vi "Main.vi"(11 "Module Admin":refnum<class "Delacor_lib_QMH_Module Admin.lvclass">) -> ()   [LabVIEW 2024, in "Aggregation 1.lvlib"]
doc: "This template is based off of the Queued Message Handler design pattern and the Queued Message Handler project template that ships with LabVIEW.\n\nThe main difference is that the queue is private to this module and communication between modules is performed via Broadcast and Request events.\n\nRequest events are wrapped in public API methods and are handled in the Event Handling Loop (EHL) of this VI. Any module can register for Broadcast events sent by this module. The EHL generates messages based on user interface actions.\n\nThe Message Handling Loop (MHL) processes messages generated by the EHL, or by other messages. The messages are string values, so new messages can be added easily to the Message Cases case structure in the MHL. Each message cluster can also provide an optional value for Message Data, which is a variant that can be converted to whatever message-specific data is required.\n_____\nBased on DQMH Dev Tools: Project Template 7.1.0.1503."
uses:
  Aggregation 1.lvlib
  <vilib>/Delacor/Delacor QMH/Libraries/Module Admin_class/Delacor_lib_QMH_Module Admin.lvclass
  Controls/Agg level 1 state cluster.ctl
  Controls/Agg level 1 state enum.ctl
  Module Data--cluster.ctl
  <vilib>/Delacor/Delacor QMH/Libraries/Message Queue_class/Delacor_lib_QMH_Message Queue.lvclass/Delacor_lib_QMH_Message Queue.ctl
  Stop Argument--cluster.ctl
  <vilib>/Delacor/Delacor QMH/Libraries/Module Admin_class/Delacor_lib_QMH_Module Admin.lvclass/Delacor_lib_QMH_Module Admin.ctl
  Serial received Argument--cluster.ctl
  Level completed Argument--cluster.ctl
  <vilib>/Utility/miscctls.llb/LVPointTypeDef.ctl
  <vilib>/Delacor/Delacor QMH/Libraries/Message Queue_class/Delacor_lib_QMH_Enqueue Message (Single).vi
  <vilib>/Delacor/Delacor QMH/Libraries/Module Admin_class/Delacor_lib_QMH_Get External Launch.vi
  <vilib>/Delacor/Delacor QMH/Libraries/Message Queue_class/Delacor_lib_QMH_Message Queue.lvclass
  DB/DB.lvlib
  GUI/GUI.lvlib
panel:
  out "error out":errorcluster
  out "Status":string
  in  "Simulate MHL Error":bool
  in  "Simulate EHL Error":bool
  # "Other processes communicate with this Module via its Public API (wrappers for its Request Events).\n\nThis Module communicates with other processes via its Broadcast Events.\nAny process that wants to receive these messages can register for this module's Broadcast events."
  # "This template is for the DQMH framework. See the block diagram for more information on how to use this template."
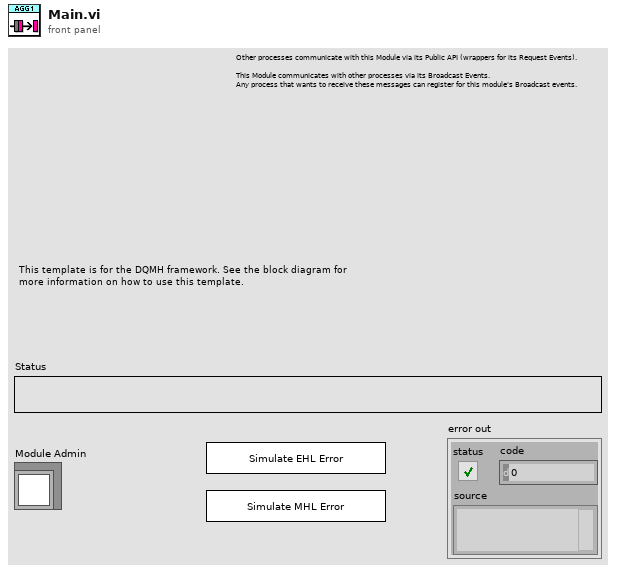
[diagram p1: front panel]
types:
  T1 = typedef "Agg level 1 state cluster.ctl" = cluster{"State":T2, "Data":variant}
  T2 = typedef "Agg level 1 state enum.ctl" = enum16{"init", "counting children", "level completed", "parent ready", "parent linked", "error", "terminate"}
  T3 = typedef "Aggregation 1.lvlib/Request Events--cluster.ctl" = cluster{"Stop Module":refnum<user-event>, "Show Panel":refnum<user-event>, "Hide Panel":refnum<user-event>, "Get Module Execution Status":refnum<user-event>, "Show Diagram":refnum<user-event>, "Serial received":refnum<user-event>, "Level completed":refnum<user-event>}
  T4 = typedef "Aggregation 1.lvlib/Module Data--cluster.ctl" = cluster{"Status":string}
  T5 = enum32{"invalid lock state", "Not Locked", "Locked (No Password)", "Password-protected"}
  T6 = typedef "Aggregation 1.lvlib/Stop Argument--cluster.ctl" = cluster{"Origin":string, "Exit via Stop Module Req?":bool, "Wait for Module to stop?":bool}
  T7 = typedef "Aggregation 1.lvlib/Serial received Argument--cluster.ctl" = cluster{"Serial":string, "index":dbl}
  T8 = typedef "Aggregation 1.lvlib/Level completed Argument--cluster.ctl" = cluster{"Serial array":string[], "Level":dbl}
  T9 = typedef "LVPointTypeDef.ctl" = cluster{"Horizontal":i16, "Vertical":i16}
  T10 = enum32{"Invalid", "Standard", "Closed", "Hidden", "Minimized", "Maximized"}
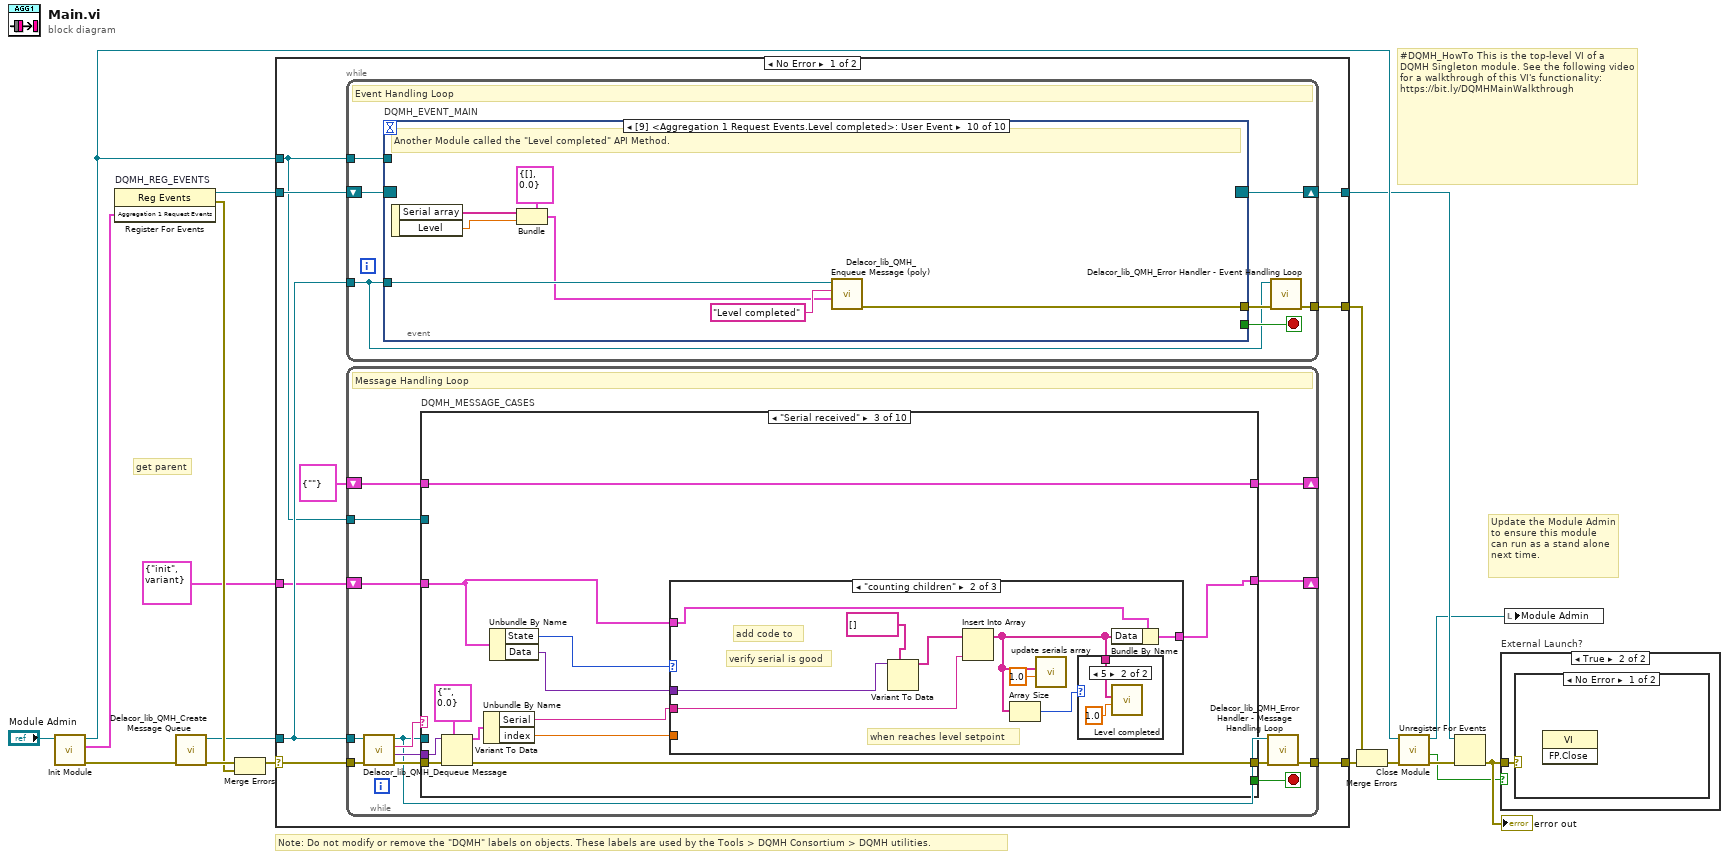
[diagram p0: block diagram]
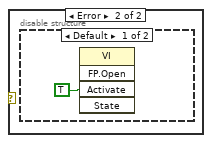
[diagram p3: hidden frame]
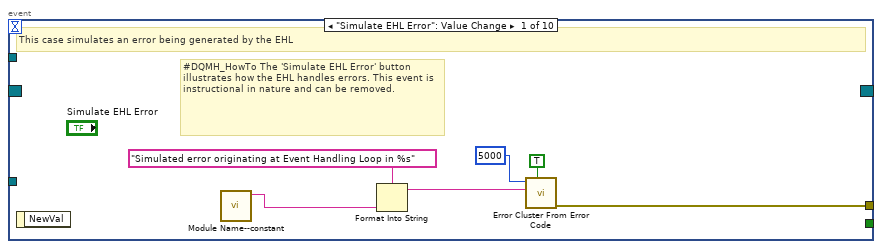
[diagram p5: hidden frame]
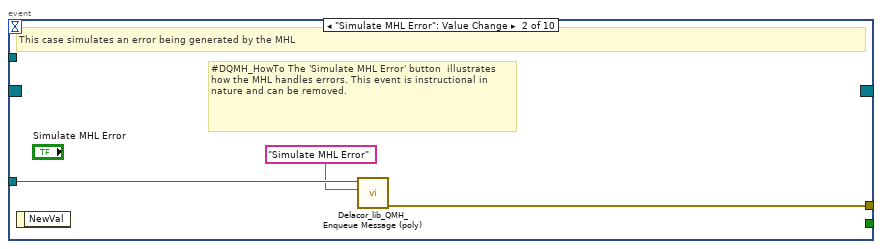
[diagram p6: hidden frame]
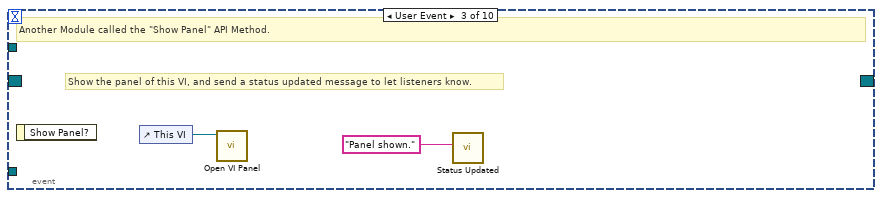
[diagram p7: hidden frame]
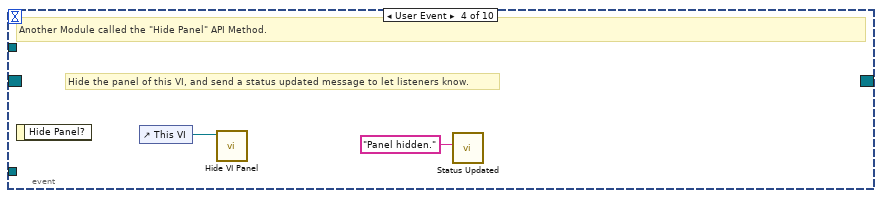
[diagram p8: hidden frame]
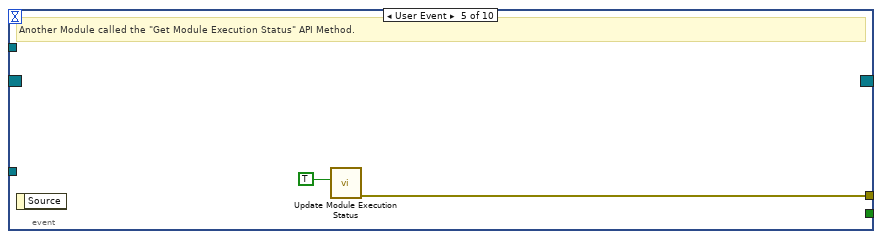
[diagram p9: hidden frame]
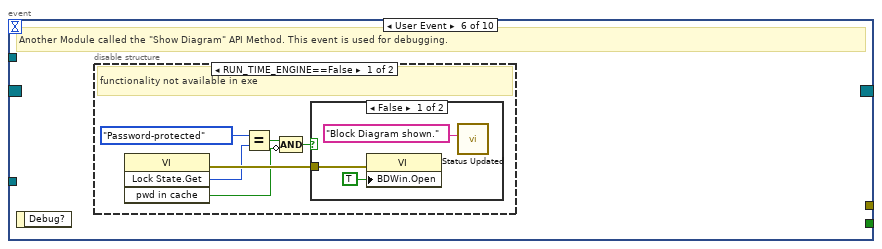
[diagram p10: hidden frame]
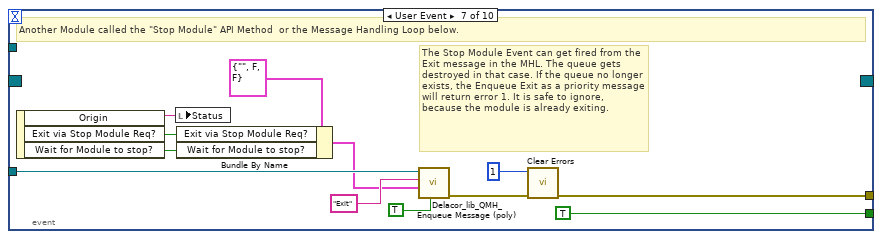
[diagram p13: hidden frame]
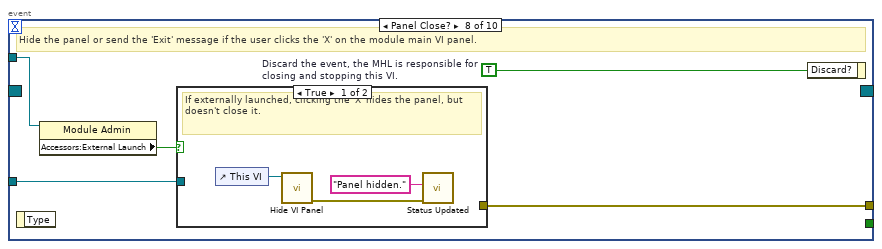
[diagram p14: hidden frame]
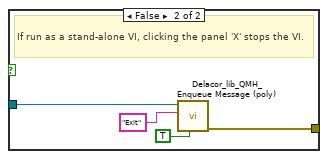
[diagram p15: hidden frame]
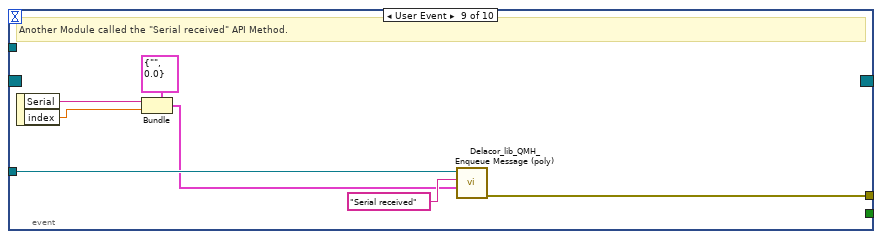
[diagram p16: hidden frame]
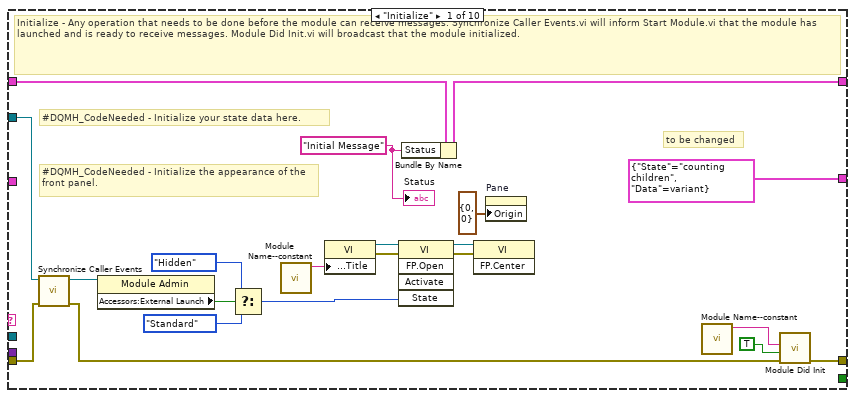
[diagram p17: hidden frame]
diagram:
  # "get parent"
  # "#DQMH_HowTo This is the top-level VI of a DQMH Singleton module. See the following video for a walkthrough of this VI's functionality: https://bit.ly/DQMHMainWalkthrough"
  # "Note: Do not modify or remove the \"DQMH\" labels on objects. These labels are used by the Tools > DQMH Consortium > DQMH utilities."
  # "Update the Module Admin to ensure this module can run as a stand alone next time."
  n1 = call "Init Module.vi"("Singleton Module Admin in"="Module Admin") -> ("error out"=w17:errorcluster, "Aggregation 1 Request Events"=w6:T3, "Singleton Module Admin out"=w9:refnum<class "Delacor_lib_QMH_Module Admin.lvclass">)  [unwired: 8 in]
  n2 = register-events "DQMH_REG_EVENTS"(w6) -> (reference out=w7:refnum<event-registration>, error out=w10:errorcluster)  [unwired: 2 in]
  n3 = call <vilib>:"Delacor_lib_QMH_Create Message Queue.vi"("error in"=w17) -> ("error out"=w12:errorcluster, "Message Queue"=w5:refnum<class "Delacor_lib_QMH_Message Queue.lvclass">)  [unwired: 9 in]
  n4 = Merge Errors(w12, w10) -> (w11:errorcluster)
  n5 = case shown="No Error" w11 {
    selector: w11 -> [w25 w248]
    tunnel: [w27 w247] -> w18
    tunnel: [w24 w246] -> w8
    tunnel: w7 -> [w22 w246]
    tunnel: w5 -> [w21 w241]
    tunnel: [w26 _] -> w15
    tunnel: w9 -> [w20 w242]
    tunnel: T1 {"State"=enum."init", "Data"=variant(dbl 0.0)} -> [w19 _]
    frame No Error {
      n6 = while {
        tunnel: w21 -> [w28]
        shift-right: [w31] -> w24
        shift-left: w22 -> [w32]
        tunnel: [w33] -> w26
        tunnel: w20 -> [w29]
        stop <- w30 stop-if-true
        # "Event Handling Loop"
        n7 = event "DQMH_EVENT_MAIN" shown="[9] <Aggregation 1 Request Events.Level completed>: User Event" {
          selector: w32 -> [_ _ _ _ _ _ _ _ _ _]
          dyn-events: [_ _ _ _ _ _ _ _ _ _] -> w31
          timeout: _ -> [_ _ _ _ _ _ _ _ _ _]
          tunnel: [_ _ _ _ _ _ TRUE ("Discard?") _ _ _] -> w30
          tunnel: w28 -> [_ w42 _ _ _ _ w66 w73 w89 w96]
          tunnel: [w40 w43 _ _ w49 _ w69 w75 w83 w90] -> w34
          tunnel: w29 -> [_ _ _ _ _ _ _ w72 _ _]
          event "Simulate EHL Error": Value Change {
            # "#DQMH_HowTo The 'Simulate EHL Error' button  illustrates how the EHL handles errors. This event is instructional in nature and can be removed."
            # "This case simulates an error being generated by the EHL"
            n8 = event-data() -> ()  [unwired: 1 in, 1 out]
            n9 = call "Module Name--constant.vi"() -> ("Module Name"=w37:string)  [unwired: 11 in]
            n10 = Format Into String(format string="Simulated error originating at Event Handling Loop in %s", w37) -> (resulting string=w38:string)  [unwired: 2 in, 1 out]
            n11 = call <vilib>:"Error Cluster From Error Code.vi"("show call chain? (False)"=TRUE, "error message (\"\")"=w38, "error code (0)"=5000) -> ("error out"=w40:errorcluster)  [unwired: 6 in]
          }
          event "Simulate MHL Error": Value Change {
            # "#DQMH_HowTo The 'Simulate MHL Error' button  illustrates how the MHL handles errors. This event is instructional in nature and can be removed."
            # "This case simulates an error being generated by the MHL"
            n12 = event-data() -> ()  [unwired: 1 in, 1 out]
            n13 = call-poly <vilib>:"Delacor_lib_QMH_Enqueue Message (poly).vi"("Message"="Simulate MHL Error", "Message Queue in"=w42) -> ("error out"=w43:errorcluster)  [unwired: 8 in, 1 out]
          }
          event User Event {
            # "Show the panel of this VI, and send a status updated message to let listeners know."
            # "Another Module called the \"Show Panel\" API Method."
            n14 = event-data() -> ()  [unwired: 1 in, 1 out]
            n15 = control-ref of="This VI"() -> (w45:refnum<vi>)
            n16 = call "Open VI Panel.vi"("VI"=w45) -> ()  [unwired: 10 in, 1 out]
            n17 = call "Status Updated.vi"("Status"="Panel shown." ("format string")) -> ()  [unwired: 10 in, 1 out]
          }
          event User Event {
            # "Hide the panel of this VI, and send a status updated message to let listeners know."
            # "Another Module called the \"Hide Panel\" API Method."
            n18 = event-data() -> ()  [unwired: 1 in, 1 out]
            n19 = control-ref of="This VI"() -> (w47:refnum<vi>)
            n20 = call "Hide VI Panel.vi"("VI"=w47) -> ()  [unwired: 10 in, 1 out]
            n21 = call "Status Updated.vi"("Status"="Panel hidden." ("format string")) -> ()  [unwired: 10 in, 1 out]
          }
          event User Event {
            # "Another Module called the \"Get Module Execution Status\" API Method."
            n22 = event-data() -> ()  [unwired: 1 in, 1 out]
            n23 = call "Update Module Execution Status.vi"("Running?"=TRUE) -> ("error out"=w49:errorcluster)  [unwired: 10 in]
          }
          event User Event {
            # "Another Module called the \"Show Diagram\" API Method. This event is used for debugging."
            n24 = event-data() -> ()  [unwired: 1 in, 1 out]
            n25 = disable-structure shown="RUN_TIME_ENGINE==False" {
              frame condition #0 (active) {
                # "functionality not available in exe"
                n26 = invoke on="Invoke Node" class="VI" method="Lock State.Get"() -> (error out=w55:errorcluster, "Get Lock State"=w54:T5, "pwd in cache"=w51:bool)  [unwired: 4 in, 1 out]
                n27 = Equal?(x=T5."Password-protected", y=w54) -> (x = y?=w52:bool)
                n28 = Compound Arithmetic op=AND(w52, invert w51) -> (w50:bool)
                n29 = case shown="False" w50 {
                  tunnel: w55 -> [w58 _]
                  frame False {
                    n30 = property on="Property Node" class="VI"(error in=w58, "BDWin.Open"=TRUE ("Block Diagram Window:Open")) -> ()  [unwired: 1 in, 2 out]
                    n31 = call "Status Updated.vi"("Status"="Block Diagram shown." ("format string")) -> ()  [unwired: 10 in, 1 out]
                  }
                  frame True {
                    # "Password-protected VI, and the password is not in the cache. Do not show the diagram."
                  }
                }
              }
              frame condition #1 {
              }
            }
          }
          event User Event {
            # "The Stop Module Event can get fired from the Exit message in the MHL. The queue gets destroyed in that case. If the queue no longer exists, the Enqueue Exit as a priority message will return error 1. It is safe to ignore, because the module is already exiting."
            # "Another Module called the \"Stop Module\" API Method  or the Message Handling Loop below."
            n32 = event-data() -> ("Origin"=w65:string, "Exit via Stop Module Req?"=w61:bool, "Wait for Module to stop?"=w60:bool)  [unwired: 1 in]
            n33 = local write "Status"(w65) -> ()
            n34 = Bundle By Name(cluster=T6 {"Origin"="", "Exit via Stop Module Req?"=FALSE, "Wait for Module to stop?"=FALSE} ("Stop Argument"), "Exit via Stop Module Req?"=w61, "Wait for Module to stop?"=w60) -> (w59:T6)
            n35 = call-poly <vilib>:"Delacor_lib_QMH_Enqueue Message (poly).vi"("Priority Message? (F)"=TRUE, "Message Data"=w59, "Message"="Exit", "Message Queue in"=w66) -> ("error out"=w70:errorcluster)  [unwired: 6 in, 1 out]
            n36 = call <vilib>:"Clear Errors.vi"("error in (no error)"=w70, "specific error code to clear (0: all)"=1) -> ("error out"=w69:errorcluster)  [unwired: 4 in, 1 out]
          }
          event Panel Close? {
            w74 = TRUE  # Discard the event, the MHL is responsible for closing and stopping this VI.
            # "Hide the panel or send the 'Exit' message if the user clicks the 'X' on the module main VI panel."
            n37 = event-data() -> ()  [unwired: 1 in, 1 out]
            n38 = property on="Property Node" class="Module Admin"(reference=w72) -> ("Accessors:External Launch"=w71:bool)  [unwired: 1 in, 2 out]
            n39 = case shown="True" w71 {
              tunnel: w73 -> [_ w81]
              tunnel: [_ w82] -> w75
              frame True {
                # "If externally launched, clicking the 'X' hides the panel, but doesn't close it."
                n40 = control-ref of="This VI"() -> (w78:refnum<vi>)
                n41 = call "Hide VI Panel.vi"("VI"=w78) -> ("error out"=w76:errorcluster)  [unwired: 10 in]
                n42 = call "Status Updated.vi"("error in"=w76, "Status"="Panel hidden." ("format string")) -> ()  [unwired: 9 in, 1 out]
              }
              frame False {
                # "If run as a stand-alone VI, clicking the panel 'X' stops the VI."
                n43 = call-poly <vilib>:"Delacor_lib_QMH_Enqueue Message (poly).vi"("Priority Message? (F)"=TRUE, "Message"="Exit", "Message Queue in"=w81) -> ("error out"=w82:errorcluster)  [unwired: 7 in, 1 out]
              }
            }
            n44 = event-data ("Event Filter Node")("Discard?"=w74) -> ()  [unwired: 1 in, 1 out]
          }
          event User Event {
            # "Another Module called the \"Serial received\" API Method."
            n45 = event-data() -> ("Serial"=w85:string, "index"=w84:dbl)  [unwired: 1 in]
            n46 = Bundle(cluster=T7 {"Serial"="", "index"=0.0} ("Serial received Argument"), "Serial"=w85, "index"=w84) -> (w86:T7)
            n47 = call-poly <vilib>:"Delacor_lib_QMH_Enqueue Message (poly).vi"("Message Data"=w86, "Message"="Serial received", "Message Queue in"=w89) -> ("error out"=w83:errorcluster)  [unwired: 7 in, 1 out]
          }
          event User Event {
            # "Another Module called the \"Level completed\" API Method."
            n48 = event-data() -> ("Serial array"=w92:string[], "Level"=w91:dbl)  [unwired: 1 in]
            n49 = Bundle(cluster=T8 {"Serial array"=[], "Level"=0.0} ("Level completed Argument"), "Serial array"=w92, "Level"=w91) -> (w93:T8)
            n50 = call-poly <vilib>:"Delacor_lib_QMH_Enqueue Message (poly).vi"("Message Data"=w93, "Message"="Level completed", "Message Queue in"=w96) -> ("error out"=w90:errorcluster)  [unwired: 7 in, 1 out]
          }
        }
        n51 = call-dynamic "Delacor_lib_QMH_Error Handler - Event Handling Loop.vi"("error in"=w34, "Message Queue in"=w28) -> ("dup error in"=w33:errorcluster)  [unwired: 8 in, 1 out]
      }
      n52 = while {
        tunnel: w21 -> [w99]
        shift-right: [w107] -> _
        shift-left: T4 {"Status"=""} ("Data Cluster") -> [w108]
        tunnel: w25 -> [w110]
        tunnel: [w102] -> w27
        tunnel: w20 -> [w103]
        shift-right: [w97] -> _
        shift-left: w19 -> [w98]
        stop <- w106 stop-if-true
        # "Message Handling Loop"
        n53 = call-dynamic "Delacor_lib_QMH_Dequeue Message.vi"("error in"=w110, "Message Queue in"=w99) -> ("error out"=w109:errorcluster, "Message Data"=w104:variant, "Message"=w105:string, "Message Queue out"=w100:refnum<class "Delacor_lib_QMH_Message Queue.lvclass">)  [unwired: 6 in]
        n54 = case "DQMH_MESSAGE_CASES" shown="\"Serial received\"" w105 {
          selector: w105 -> [_ _ _ _ _ _ _ _ _ w236]
          tunnel: w100 -> [_ _ _ _ _ _ _ w200 w223 _]
          tunnel: w109 -> [w129 w134 w146 w173 w182 w185 w195 w207 w229 w239]
          tunnel: [w127 w134 w144 w171 w181 w185 w194 w203 w224 w240] -> w101
          tunnel: w108 -> [w118 w133 w145 w172 w180 w184 w192 w202 w222 w237]
          tunnel: [w117 w133 w145 w172 w180 w184 w192 w202 w222 w237] -> w107
          tunnel: [_ _ _ _ _ _ _ _ w221 _] -> w106
          tunnel: w104 -> [_ _ w143 w170 _ _ _ w201 w220 _]
          tunnel: w103 -> [w119 _ _ _ _ _ _ w199 w215 _]
          tunnel: w98 -> [_ w132 w135 w160 w179 w183 w186 w196 w214 w230]
          tunnel: [T1 {"State"=enum."counting children", "Data"=variant} w132 w136 w161 w179 w183 w186 w196 w214 w230] -> w97
          frame "Initialize" {
            w113 = "Initial Message" ("Initial Message")
            # "to be changed"
            # "#DQMH_CodeNeeded - Initialize the appearance of the front panel."
            # "#DQMH_CodeNeeded - Initialize your state data here."
            # "Initialize - Any operation that needs to be done before the module can receive messages. Synchronize Caller Events.vi will inform Start Module.vi that the module has launched and is ready to receive messages. Module Did Init.vi will broadcast that the module initialized."
            n55 = call "Synchronize Caller Events.vi"("error in"=w129, "Singleton Module Admin in"=w119) -> ("error out"=w128:errorcluster, "Singleton Module Admin out"=w114:refnum<class "Delacor_lib_QMH_Module Admin.lvclass">)  [unwired: 8 in]
            n56 = property on="Property Node" class="Module Admin"(reference=w114) -> ("Accessors:External Launch"=w123:bool)  [unwired: 1 in, 2 out]
            n57 = Select(t=T10."Hidden" ("State"), s=w123, f=T10."Standard" ("State")) -> (s? t:f=w120:T10)
            n58 = call "Module Name--constant.vi"() -> ("Module Name"=w126:string)  [unwired: 11 in]
            n59 = property on="Property Node" class="VI"("Front Panel.Title"=w126) -> (reference out=w125:refnum<vi>, error out=w131:errorcluster)  [unwired: 2 in]
            n60 = invoke on="Invoke Node" class="VI" method="FP.Open"(reference=w125, error in=w131, "State"=w120) -> (reference out=w124:refnum<vi>, error out=w130:errorcluster)  [unwired: 2 in, 3 out]
            n61 = Bundle By Name(cluster=w118, "Status"=w113) -> (w117:T4)
            n62 = invoke on="Invoke Node" class="VI" method="FP.Center"(reference=w124, error in=w130) -> ()  [unwired: 1 in, 3 out]
            n63 = property on="Pane" class="Pane"("Origin"=T9 {"Horizontal"=0, "Vertical"=0}) -> ()  [unwired: 2 in, 2 out]
            n64 = call "Module Name--constant.vi"() -> ("Module Name"=w115:string)  [unwired: 11 in]
            n65 = call "Module Did Init.vi"("error in"=w128, "Initialized?"=TRUE, "Origin"=w115) -> ("error out"=w127:errorcluster)  [unwired: 8 in]
            "Status" <- w113
          }
          frame "---Module Specific---" {
            # "Separator -- The following cases handle messages specific to this Module."
          }
          frame "Serial received" {
            n66 = Variant To Data(error in=w146, type=T7 {"Serial"="", "index"=0.0} ("Serial received Argument"), Variant=w143) -> (data=w141:T7, error out=w144:errorcluster)
            n67 = Unbundle By Name(w141) -> ("Serial"=w139:string, "index"=w137:dbl)
            n68 = Unbundle By Name(w135) -> ("State"=w140:T2, "Data"=w138:variant)
            n69 = case shown="\"counting children\"" w140 {
              tunnel: w139 -> [_ w153 _]
              tunnel: w138 -> [_ w156 _]
              tunnel: w137 -> [_ _ _]
              tunnel: [w147 w152 w159] -> w136
              tunnel: w135 -> [w147 w151 w159]
              frame "init", Default {
              }
              frame "counting children" {
                # "when reaches level setpoint"
                # "add code to"
                # "verify serial is good"
                n70 = Variant To Data(type=string[] [], Variant=w156) -> (data=w154:string[])  [unwired: 1 in, 1 out]
                n71 = Insert Into Array(array=w154, new element=w153) -> (w149:string[])  [unwired: 1 in]
                n72 = Array Size(array=w149) -> (size(s)=w150:i32)
                n73 = call "update serials array.vi"("level"=1.0, "serial array"=w149) -> ()  [unwired: 9 in, 1 out]
                n74 = case shown="5" w150 {
                  tunnel: w149 -> [_ w158]
                  frame 0, Default {
                  }
                  frame 5 {
                    n75 = call "Level completed.vi"("Level"=1.0, "Serial array"=w158) -> ()  [unwired: 9 in, 1 out]
                  }
                }
                n76 = Bundle By Name(cluster=w151, "Data"=w149) -> (w152:T1)
              }
              frame "level completed" {
              }
            }
          }
          frame "Level completed" {
            n77 = Variant To Data(error in=w173, type=T8 {"Serial array"=[], "Level"=0.0} ("Level completed Argument"), Variant=w170) -> (data=w168:T8, error out=w171:errorcluster)
            n78 = Unbundle By Name(w168) -> ("Serial array"=w167:string[], "Level"=w162:dbl)
            n79 = call "get parent.vi"("Level number"=w162) -> ("timed out?"=w164:bool, "Parent"=w166:string)  [unwired: 8 in, 1 out]
            n80 = Empty String/Path?(string/path=w166) -> (empty?=w165:bool)
            n81 = Or(x=w165, y=w164) -> (x .or. y?=w163:bool)
            n82 = case shown="False" w163 {
              tunnel: w166 -> [w176 _]
              tunnel: w167 -> [w177 _]
              tunnel: w162 -> [w175 _]
              tunnel: [T1 {"State"=enum."counting children", "Data"=variant} w178] -> w161
              tunnel: w160 -> [_ w178]
              frame False {
                # "response received"
                n83 = call "link parent to children.vi"("Parent"=w176, "Serial array"=w177, "Level"=w175) -> ()  [unwired: 8 in, 1 out]
                n84 = call "update parent.vi"("level"=w175, "Parent"=w176) -> ()  [unwired: 9 in, 1 out]
              }
              frame True {
                # "Time out or empty prent"
              }
            }
          }
          frame "---Copy This Frame---" {
            # "Duplicate this frame when creating new messages.  Change this comment in the duplicated frame to describe this message."
            n85 = Merge Errors(w182) -> (w181:errorcluster)
          }
          frame "---Exit and Error Handling---" {
            # "Separator - The following cases handle errors and exit messages."
          }
          frame "Simulate MHL Error" {
            # "#DQMH_HowTo The 'Simulate MHL Error' button  illustrates how the MHL handles errors. This event is instructional in nature and can be removed."
            # "Simulate an error occurring at the MHL"
            n86 = call "Module Name--constant.vi"() -> ("Module Name"=w188:string)  [unwired: 11 in]
            n87 = Format Into String(format string="Simulated error originating at Message Handling Loop in %s", w188) -> (resulting string=w189:string)  [unwired: 2 in, 1 out]
            n88 = call <vilib>:"Error Cluster From Error Code.vi"("show call chain? (False)"=TRUE, "error message (\"\")"=w189, "error code (0)"=5001) -> ("error out"=w193:errorcluster)  [unwired: 6 in]
            n89 = Merge Errors(w195, w193) -> (w194:errorcluster)
          }
          frame "Error" {
            # "#DQMH_CodeRecommended - If the module is running in standalone mode (External Launch = FALSE), this code will pop up an error dialog and call the 'Exit' message if an error occurs. Add more fine-grained error management here."
            # "Error - Check the error message data and respond accordingly. This message is sent by the \"Error Handler\" VIs at the end of each loop in this application."
            n90 = property on="Property Node" class="Module Admin"(reference=w199) -> ("Accessors:External Launch"=w198:bool)  [unwired: 1 in, 2 out]
            n91 = Variant To Data(error in=w207, type=errorcluster {"status"=FALSE, "code"=0, "source"=""} ("error constant"), Variant=w201) -> (data=w197:errorcluster, error out=w205:errorcluster)
            n92 = local write "error out"(w197) -> ()
            n93 = call "Error Reported.vi"("Error"=w197) -> ()  [unwired: 10 in, 1 out]
            n94 = case shown="False" w198 {
              tunnel: [w212 _] -> w204
              tunnel: w200 -> [w210 _]
              tunnel: w197 -> [w211 _]
              frame False {
                n95 = disable-structure shown="Default" {
                  disable-tunnel: w211 -> [w213 _]
                  frame condition #0 (active) {
                    # "If the module is running standalone, then pop up an error dialog and call the \"Exit\" message."
                    n96 = call <vilib>:"Simple Error Handler.vi"("error in (no error)"=w213) -> ()  [unwired: 4 in, 5 out]
                  }
                  frame condition #1 {
                    # "To prevent the Simple Error Handler VI from being loaded (e.g. when deploying to a Real-Time target), add the Conditional Disable Symbol \"DQMH_Disable_SEH\" to your project and set it to TRUE."
                  }
                }
                n97 = call-poly <vilib>:"Delacor_lib_QMH_Enqueue Message (poly).vi"("Priority Message? (F)"=TRUE, "Message"="Exit", "Message Queue in"=w210) -> ("error out"=w212:errorcluster)  [unwired: 7 in, 1 out]
              }
              frame True {
                # "If the module was launched externally, calling the Error Reported broadcast VI is the only action performed by the \"Error\" message. The module's caller can then process the error appropriately."
              }
            }
            n98 = Merge Errors(w205, w204) -> (w203:errorcluster)
          }
          frame "Exit" {
            w219 = 91  # 91: not all Exit messages will have an argument
            w221 = TRUE  # Stop the VI
            # "Release the message queue reference"
            # "#DQMH_CodeNeeded - Add any required cleanup code here."
            # "Exit - Exit the application."
            n99 = Variant To Data(error in=w229, type=T6 {"Origin"="", "Exit via Stop Module Req?"=FALSE, "Wait for Module to stop?"=FALSE} ("Stop Argument"), Variant=w220) -> (data=w217:T6, error out=w226:errorcluster)
            n100 = call <vilib>:"Clear Errors.vi"("error in (no error)"=w226, "specific error code to clear (0: all)"=w219) -> ("error out"=w228:errorcluster)  [unwired: 4 in, 1 out]
            n101 = control-ref of="This VI"() -> (w216:refnum<vi>)
            n102 = call-dynamic "Delacor_lib_QMH_Release Message Queue.vi"("error in"=w228, "Message Queue"=w223) -> ("error out"=w227:errorcluster)  [unwired: 9 in]
            n103 = call "Handle Exit.vi"("Stop Argument"=w217, "Admin in"=w215, "VI reference"=w216) -> ("error out"=w225:errorcluster)  [unwired: 7 in, 1 out]
            n104 = Merge Errors(w227, w225) -> (w224:errorcluster)
            n105 = call "Error Reported.vi"("Error"=w224) -> ()  [unwired: 10 in, 1 out]
          }
          frame Default {
            # "'Default' case only runs if there is a message that isn't defined in any of the other cases.  Output a programming error."
            n106 = call "Module Name--constant.vi"() -> ("Module Name"=w235:string)  [unwired: 11 in]
            n107 = Format Into String(format string="The invalid message string \"%s\" was received in the Message Handling Loop for module \"%s\".", w236, w235) -> (resulting string=w231:string)  [unwired: 2 in, 1 out]
            n108 = call <vilib>:"Error Cluster From Error Code.vi"("show call chain? (False)"=TRUE, "error message (\"\")"=w231, "error code (0)"=1) -> ("error out"=w238:errorcluster)  [unwired: 6 in]
            n109 = Merge Errors(w239, w238) -> (w240:errorcluster)
          }
        }
        n110 = call-dynamic "Delacor_lib_QMH_Error Handler - Message Handling Loop.vi"("error in"=w101, "Message Queue in"=w100) -> ("dup error in"=w102:errorcluster)  [unwired: 8 in, 1 out]
      }
    }
    frame Error {
      # "Synchronize Caller Events.vi will inform Start Module.vi that the module has launched and will let the code calling Start Module.vi register for broadcasts and would permit the caller receive the broadcast that an error occurred at launch time."
      n111 = call-dynamic "Delacor_lib_QMH_Release Message Queue.vi"("error in"=w248, "Message Queue"=w241) -> ("error out"=w247:errorcluster)  [unwired: 9 in]
      n112 = call "Synchronize Caller Events.vi"("Singleton Module Admin in"=w242) -> ("error out"=w249:errorcluster)  [unwired: 9 in, 1 out]
      n113 = call "Module Name--constant.vi"() -> ("Module Name"=w245:string)  [unwired: 11 in]
      n114 = Format Into String(format string="An error occurred during initialization. %s is no longer running.", w245) -> (resulting string=w243:string)  [unwired: 2 in, 1 out]
      n115 = Merge Errors(w247, w249) -> (w250:errorcluster)
      n116 = call "Error Reported.vi"("Additional Information"=w243, "Error"=w250) -> ()  [unwired: 9 in, 1 out]
    }
  }
  n117 = Merge Errors(w15, w18) -> (w14:errorcluster)
  n118 = call "Close Module.vi"("error in"=w14, "Module Admin in"=w9) -> ("error out"=w16:errorcluster, "External Launch"=w2:bool, "Module Admin out"=w3:refnum<class "Delacor_lib_QMH_Module Admin.lvclass">)  [unwired: 7 in]
  n119 = Unregister For Events(event registration refnum=w8, error in=w16) -> (error out=w13:errorcluster)
  "error out" <- w13
  n120 = case "External Launch?" shown="True" w2 {
    tunnel: w13 -> [_ w251]
    frame False {
    }
    frame True {
      n121 = case shown="No Error" w251 {
        frame No Error {
          n122 = invoke on="Invoke Node" class="VI" method="FP.Close"() -> ()  [unwired: 3 in, 3 out]
        }
        frame Error {
          n123 = disable-structure shown="Default" {
            frame condition #0 (active) {
              n124 = invoke class="VI" method="FP.Open"("Activate"=TRUE ("Activate?")) -> ()  [unwired: 4 in, 5 out]
            }
            frame condition #1 {
              # "Don't show panel on error if running inside a built EXE."
            }
          }
        }
      }
    }
  }
  n125 = local write "Module Admin"(w3) -> ()
